vi "Acquire_Prototype.vi"() -> ()   [LabVIEW 2013, in "MagSpec_Bella.lvclass"]
uses:
  MagSpec_Bella.lvclass
  Controls/CamAndObj_TypDEf_Bella.ctl
  Controls/ScreenCam2_TypDEf_Bella.ctl
  MagSpec_Bella.lvclass/MagSpec_Bella.ctl
  <vilib>/vision/NI_Vision_Development_Module.lvlib
panel:
  out "get Images":u32
  out "Array 3":i32[][](array[numeric])
  out "Array 2":i32[][](array[numeric])
  out "time":u32[](array[numeric])
  out "total time":u32
  out "B":dbl
  in  "Sim Image Index 2":i32=3
  in  "B [T] in":dbl=0.63
  out "Numeric 3":i32
  in  "stop":bool
  out "Image Out":T1(plugin-control)
  out "Empty Image":bool[](array[boolean])
  out "error out":errorcluster
  out "Sum Y":cluster{"Momentum [MeV/C]":dbl[], dbl[]}[](graph)
  in  "MagSpec_Bella.lvclass":refnum<class "MagSpec_Bella.lvclass">
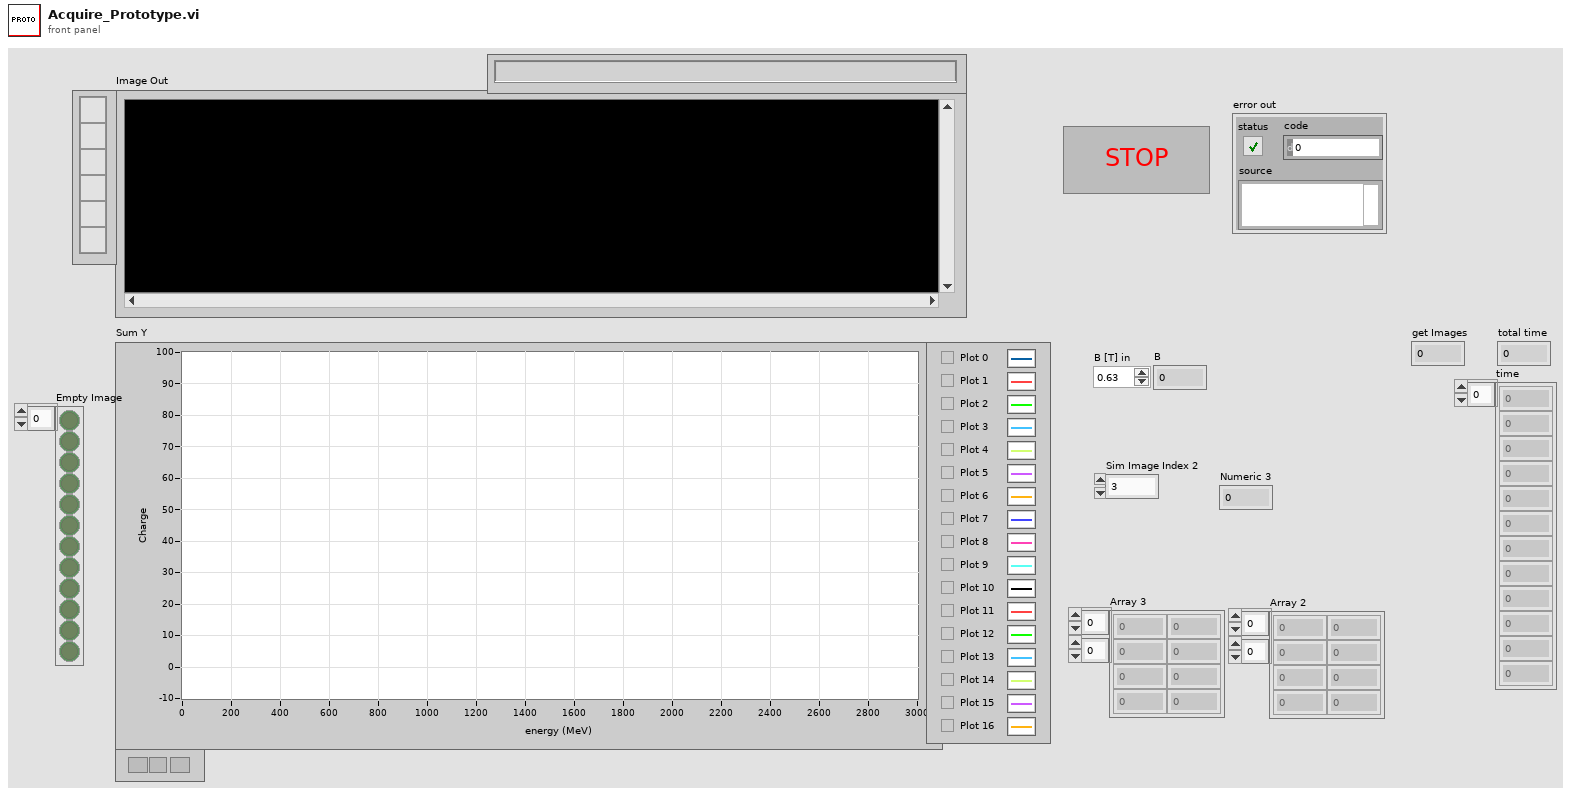
[diagram p1: front panel]
types:
  T1 = typedef "IMAQ Image.ctl" = refnum<image>
  T2 = typedef "Image Type" = u32
  T3 = typedef "CameraSettings_File.ctl" = cluster{"FOV [mm]":dbl, "Left edge [mm]":dbl, "ROI Y offset":dbl, "ROI height":dbl, "ROI X offset":dbl, "ROI width":dbl, "Y center pixel":dbl, "Y Start":dbl, "Y End":dbl, "X Start":dbl, "X End":dbl, "rot [deg]":dbl}
  T4 = typedef "ScreenCam2_TypDEf_Bella.ctl" = cluster{"Screen Orientation":string, "Screen angle":string, "Lens":T5, "Calibration (mm/pix)":dbl}
  T5 = typedef "CamAndObj_TypDEf_Bella.ctl" = enum16{"FL1-f8x08", "FL1-f8x06", "FL1-f8", "ch300-f50", "FL2G-f8", "FL3M14-f8", "FL3M14-f8x08", "FL3M14-f8x08(2x2)"}
  T6 = cluster{"npix-X":i32, "npix-Y":i32, "Left [pix]":dbl, "Top [pix]":dbl}
  T7 = typedef "OneTimeCalculation.ctl" = cluster{"first Pixel pos [m]":dbl, "Pixel Size [mm]":dbl, "forward":T8}
  T8 = typedef "OnOffTypeDef.ctl" = enum16{"off", "on"}
  T9 = typedef "2D.ctl" = cluster{"dp":dbl[][], "chargeCompensation":dbl[][], "angle":dbl[][], "Momentum":dbl[][]}
  T10 = typedef "finalCalib--Cluster.ctl" = cluster{"X":dbl[][], "xi":dbl[][], "delta momentum":dbl, "Y":dbl[][], "yi":dbl[][], "angle (Y)":dbl[], "delta angle":dbl, "scale delta angle":dbl, "intraX":dbl, "intraY":dbl, "mask":dbl[][]}
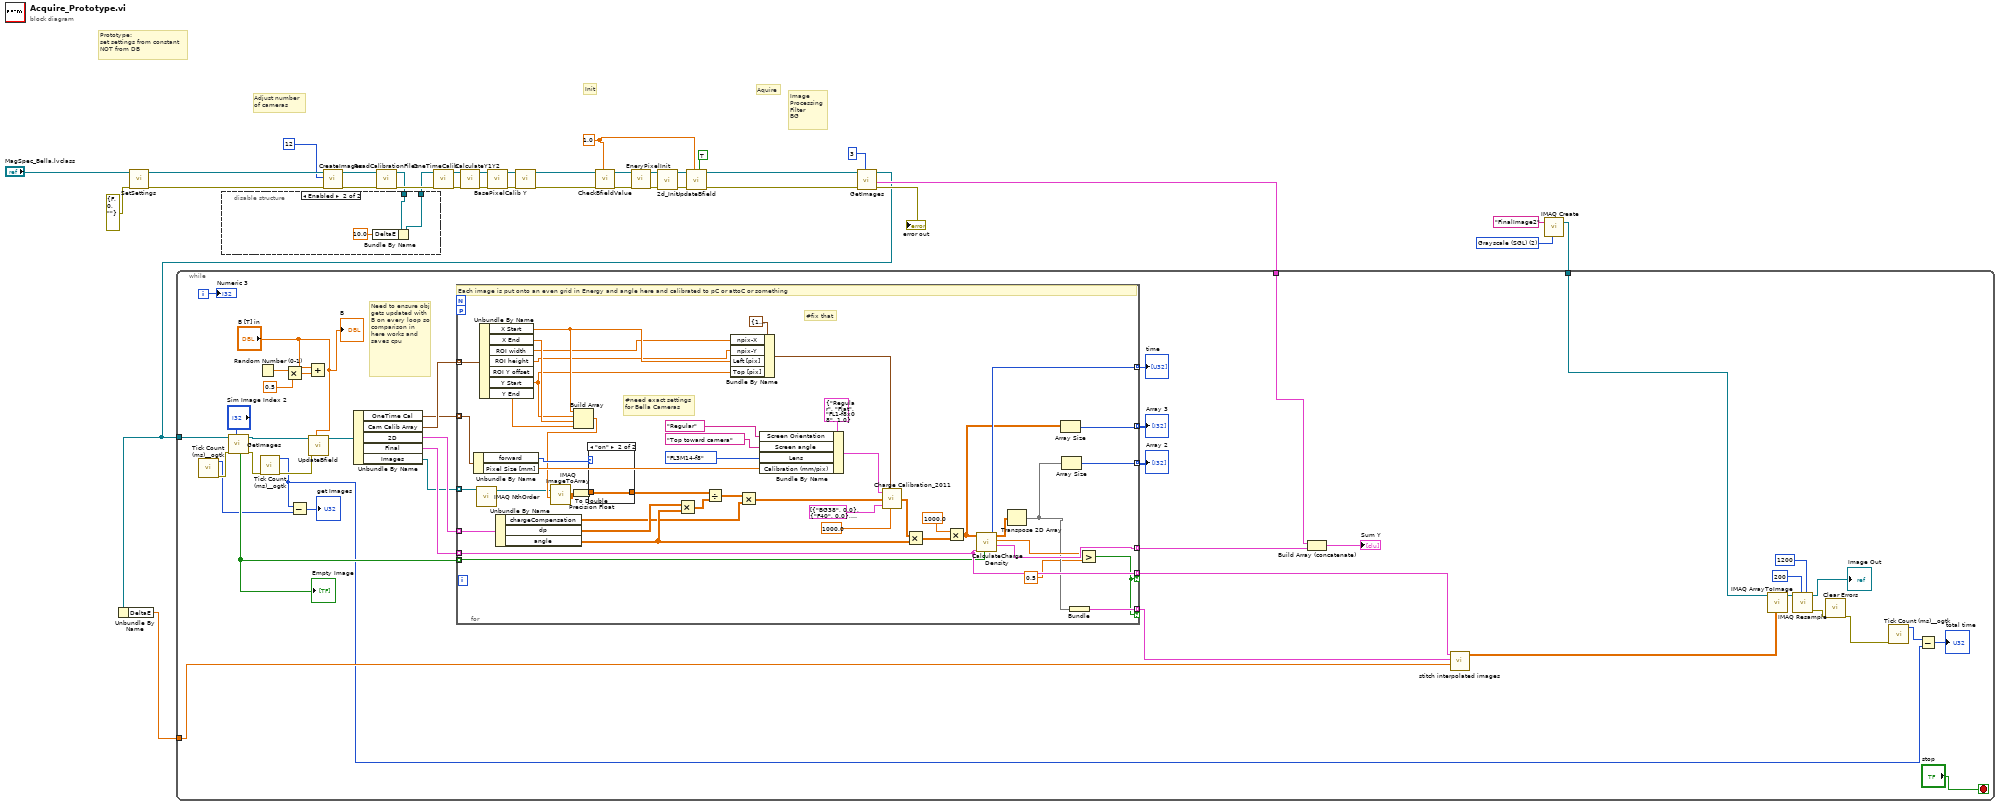
[diagram p0: block diagram]
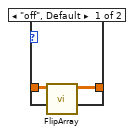
[diagram p2: hidden frame]
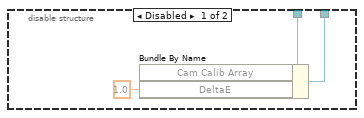
[diagram p3: hidden frame]
diagram:
  w3 = 1.0 ("B [T] in")
  w7 = T2 2 items=["Grayscale (U8)", "Grayscale (I16)", "Grayscale (SGL)", "Complex (CSG)", "RGB (U32)", "HSL (U32)", "RGB (U64)", "Grayscale (U16)"] ("Image Type")
  # "Image\nProcessing\nFilter\nBG"
  # "Adjust number\nof cameras"
  # "Aquire"
  # "Init"
  # "Prototype:\nset settings from constant\nNOT from DB"
  n1 = call "SetSettings.vi"("error in (no error)"=errorcluster {"status"=FALSE, "code"=0, "source"=""} ("error out"), "MagSpec_Bella in"="MagSpec_Bella.lvclass") -> ("error out"=w31:errorcluster, "MagSpec_Bella out"=w33:refnum<class "MagSpec_Bella.lvclass">)  [unwired: 8 in]
  n2 = call "CreateImages.vi"("error in (no error)"=w31, "Numeric"=12, "MagSpec_Bella in"=w33) -> ("error out"=w30:errorcluster, "MagSpec_Bella out"=w15:refnum<class "MagSpec_Bella.lvclass">)  [unwired: 7 in]
  n3 = call "ReadCalibrationFiles.vi"("error in (no error)"=w30, "MagSpec_Bella in"=w15) -> ("error out"=w29:errorcluster, "MagSpec_Bella out"=w14:refnum<class "MagSpec_Bella.lvclass">)  [unwired: 8 in]
  n4 = disable-structure shown="Enabled" {
    disable-tunnel: w14 -> [w38 w42]
    disable-tunnel: [w37 w41] -> w13
    frame Disabled {
      n5 = Bundle By Name(cluster=w38, "DeltaE"=1.0) -> (w37:refnum<class "MagSpec_Bella.lvclass">, "Cam Calib Array"=w39:T3[])
    }
    frame Enabled {
      n6 = Bundle By Name(cluster=w42, "DeltaE"=10.0) -> (w41:refnum<class "MagSpec_Bella.lvclass">)
    }
  }
  n7 = call "OneTimeCalib.vi"("error in"=w29, "MagSpec_Bella in"=w13) -> ("error out"=w24:errorcluster, "MagSpec_Bella out"=w25:refnum<class "MagSpec_Bella.lvclass">)  [unwired: 8 in]
  n8 = call "CalculateY1Y2.vi"("error in"=w24, "MagSpec_Bella in"=w25) -> ("error out"=w22:errorcluster, "MagSpec_Bella out"=w23:refnum<class "MagSpec_Bella.lvclass">)  [unwired: 8 in]
  n9 = call "BasePixelCalib.vi"("error in (no error)"=w22, "MagSpec_Bella in"=w23) -> ("error out"=w19:errorcluster, "MagSpec_Bella out"=w21:refnum<class "MagSpec_Bella.lvclass">)  [unwired: 8 in]
  n10 = call "Y.vi"("error in (no error)"=w19, "MagSpec_Bella in"=w21) -> ("error out"=w18:errorcluster, "MagSpec_Bella out"=w20:refnum<class "MagSpec_Bella.lvclass">)  [unwired: 8 in]
  n11 = call "CheckBfieldValue .vi"("B [T] new"=w3, "MagSpec_Bella in"=w20) -> ("MagSpec_Bella out"=w8:refnum<class "MagSpec_Bella.lvclass">)  [unwired: 8 in, 1 out]
  n12 = call "EneryPixelInit.vi"("error in (no error)"=w18, "MagSpec_Bella in"=w8) -> ("error out"=w9:errorcluster, "MagSpec_Bella out"=w10:refnum<class "MagSpec_Bella.lvclass">)  [unwired: 8 in]
  n13 = call "2d_Init.vi"("error in (no error)"=w9, "MagSpec_Bella in"=w10) -> ("error out"=w26:errorcluster, "MagSpec_Bella out"=w27:refnum<class "MagSpec_Bella.lvclass">)  [unwired: 8 in]
  n14 = call "UpdateBfield.vi"("Force upodate (F)"=TRUE ("Force upodate"), "B [T] in"=w3, "error in (no error)"=w26, "MagSpec_Bella in"=w27) -> ("error out"=w28:errorcluster, "MagSpec_Bella out"=w35:refnum<class "MagSpec_Bella.lvclass">)  [unwired: 6 in]
  n15 = call "GetImages.vi"("Sim Image Index"=3, "error in (no error)"=w28, "MagSpec_Bella in"=w35) -> ("error out"=→"error out":errorcluster, "output cluster"=w12:cluster{dbl[], dbl[]}[], "MagSpec_Bella out"=w2:refnum<class "MagSpec_Bella.lvclass">)  [unwired: 5 in, 1 out]
  n16 = Unbundle By Name(w2) -> ("DeltaE"=w1:dbl)
  n17 = call "IMAQ Create"("Image Name"="FinalImage2", "Image Type"=w7) -> ("New Image"=w5:T1)  [unwired: 3 in, 1 out]
  n18 = while {
    tunnel: w12 -> [w78]
    tunnel: w5 -> [w77]
    tunnel: w2 -> [w66]
    tunnel: w1 -> [w60]
    i -> [w71]
    stop <- "stop" stop-if-true
    # "Need to ensure obj gets updated with B on every loop so comparison in here works and saves cpu"
    n19 = call <userlib>:"Tick Count (ms)__ogtk.vi"() -> ("error out"=w46:errorcluster, "millisecond timer value"=w44:u32)  [unwired: 10 in]
    n20 = call "GetImages.vi"("Sim Image Index"="Sim Image Index 2", "error in (no error)"=w46, "MagSpec_Bella in"=w66) -> ("error out"=w48:errorcluster, "MagSpec_Bella out"=w65:refnum<class "MagSpec_Bella.lvclass">, "Empty Image"=w58:bool[])  [unwired: 5 in, 1 out]
    "Empty Image" <- w58
    n21 = Random Number (0-1)() -> (number: 0 to 1=w70:dbl)
    n22 = call <userlib>:"Tick Count (ms)__ogtk.vi"("error in (no error)"=w48) -> ("error out"=w47:errorcluster, "millisecond timer value"=w45:u32)  [unwired: 9 in]
    n23 = Multiply(x=w70, y=0.5) -> (x*y=w68:dbl)
    n24 = Subtract(x=w45, y=w44) -> (x-y=→"get Images":u32)
    n25 = Add(x="B [T] in", y=w68) -> ()  [unwired: 1 out]
    n26 = call "UpdateBfield.vi"("B [T] in"="B [T] in", "error in (no error)"=w47, "MagSpec_Bella in"=w65) -> ("MagSpec_Bella out"=w73:refnum<class "MagSpec_Bella.lvclass">)  [unwired: 7 in, 1 out]
    n27 = Unbundle By Name(w73) -> ("OneTime Cal"=w79:T7[], "Cam Calib Array"=w80:T3[], "2D"=w83:T9[], "Final"=w82:T10[], "Images"=w81:T1[])
    n28 = for {
      tunnel: w83 -> [w131] mode=indexing
      tunnel: w82 -> [w96] mode=indexing
      tunnel: w81 -> [w116] mode=indexing
      tunnel: w80 -> [w129] mode=indexing
      tunnel: w79 -> [w128] mode=indexing
      tunnel: [w117] -> w76 mode=indexing
      tunnel: [w96] -> w75 mode=indexing if=w93
      tunnel: [w95] -> w74 mode=indexing if=w93
      workers-P: _ -> [_]
      tunnel: w58 -> [w90] mode=indexing
      tunnel: [w89] -> w49 mode=indexing
      tunnel: [w87] -> w62 mode=indexing
      tunnel: [w85] -> w61 mode=indexing
      # "#fix that"
      # "#need exact settings\nfor Bella Cameras"
      # "Each image is put onto an even grid in Energy and angle here and calibrated to pC or attoC or something"
      n29 = Unbundle By Name(w128) -> ("forward"=w103:T8, "Pixel Size [mm]"=w127:dbl)
      n30 = call "IMAQ NthOrder"("Image Src"=w116) -> ("Image Dst Out"=w101:T1)  [unwired: 6 in, 1 out]
      n31 = Unbundle By Name(w129) -> ("X Start"=w107:dbl, "X End"=w112:dbl, "ROI width"=w105:dbl, "ROI height"=w104:dbl, "Y Start"=w106:dbl, "Y End"=w111:dbl)  [unwired: 1 out]
      n32 = Unbundle By Name(w131) -> ("chargeCompensation"=w114:dbl[][], "dp"=w115:dbl[][], "angle"=w130:dbl[][])
      n33 = Build Array(w107, w106, w112, w111) -> (w102:dbl[])
      n34 = call "IMAQ ImageToArray"("Optional Rectangle"=w102, "Image"=w101) -> ("Image Pixels (Float)"=w97:sgl[][])  [unwired: 2 in, 4 out]
      n35 = To Double Precision Float(number=w97) -> (double precision float=w109:dbl[][])
      n36 = case shown="\"on\"" w103 {
        tunnel: w109 -> [w133 w134]
        tunnel: [w132 w134] -> w108
        frame "off", Default {
          n37 = call "FlipArray.vi"("In"=w133) -> ("Out"=w132:dbl[][])  [unwired: 10 in]
        }
        frame "on" {
        }
      }
      n38 = Multiply(x=w115, y=w130) -> (x*y=w92:dbl[][])
      n39 = Divide(x=w108, y=w92) -> (x/y=w91:dbl[][])
      n40 = Bundle By Name(cluster=T6 {"npix-X"=1384, "npix-Y"=300, "Left [pix]"=0.0, "Top [pix]"=0.0} ("ROI infos"), "npix-X"=w105, "npix-Y"=w104, "Left [pix]"=w107, "Top [pix]"=w106) -> (w98:T6)
      n41 = Multiply(x=w91, y=w114) -> (x*y=w113:dbl[][])
      n42 = Bundle By Name(cluster=T4 {"Screen Orientation"="Regular", "Screen angle"="Flat", "Lens"=enum."FL1-f8x08", "Calibration (mm/pix)"=1.0} ("Screen&Camera 2"), "Screen Orientation"="Regular", "Screen angle"="Top toward camera", "Lens"=CamAndObj_TypDEf_Bella."FL3M14-f8", "Calibration (mm/pix)"=w127) -> (w122:T4)
      n43 = call "Charge Calibration_2011.vi"("Screen&Camera 2"=w122, "ROI infos"=w98, "Image (Counts)"=w113, "Filters"=cluster{"Name":string, "#Filters":dbl}[] [{"Name"="BG38", "#Filters"=0.0}, {"Name"="F40", "#Filters"=0.0}, {"Name"="F70", "#Filters"=1.0}, {"Name"="oldBP", "#Filters"=0.0}], "Electron energy (MeV)"=1000.0) -> ("Image (pC)"=w120:dbl[][])  [unwired: 4 in]
      n44 = Multiply(x=w120, y=w130) -> (x*y=w100:dbl[][])
      n45 = Multiply(x=1000.0, y=w100) -> (x*y=w86:dbl[][])
      n46 = call "CalculateChargeDensity.vi"("empty image"=w90, "Final"=w96, "Z"=w86) -> ("spec cluster 2"=w117:cluster{"Momentum [MeV/C]":dbl[], dbl[]}, "charge (sum)"=w94:dbl, "charge density"=w118:dbl[][], "time: 2Dinter"=w89:u32)  [unwired: 4 in, 1 out]
      n47 = Transpose 2D Array(2D array=w118) -> (transposed array=w88:dbl[][])
      n48 = Array Size(array=w86) -> (size(s)=w85:i32[])
      n49 = Array Size(array=w88) -> (size(s)=w87:i32[])
      n50 = Bundle(w88) -> (w95:cluster{dbl[][]})  [unwired: 1 in]
      n51 = Greater?(x=w94, y=0.5 ("change threshold")) -> (0:w93:bool)
    }
    "time" <- w49
    "Array 2" <- w62
    "Array 3" <- w61
    n52 = Build Array (concatenate)(w78, w76) -> (→"Sum Y":cluster{"Momentum [MeV/C]":dbl[], dbl[]}[])
    n53 = call "stitch interpolated images.vi"("DeltaE"=w60, "Array of images to stitch"=w74, "calib \"final\""=w75) -> ("stitched array image"=w55:sgl[][])  [unwired: 8 in]
    n54 = call "IMAQ ArrayToImage"("Image Pixels (Float)"=w55, "Image"=w77) -> ("Image Out"=w54:T1)  [unwired: 8 in, 1 out]
    n55 = call "IMAQ Resample"("X Resolution"=1200, "Y Resolution"=200, "Image Src"=w54) -> ("error out"=w51:errorcluster, "Image Dst Out"=→"Image Out":T1)  [unwired: 7 in]
    n56 = call <vilib>:"Clear Errors.vi"("error in (no error)"=w51) -> ("error out"=w63:errorcluster)  [unwired: 6 in]
    n57 = call <userlib>:"Tick Count (ms)__ogtk.vi"("error in (no error)"=w63) -> ("millisecond timer value"=w57:u32)  [unwired: 9 in, 1 out]
    n58 = Subtract(x=w57, y=w45) -> (x-y=→"total time":u32)
    "Numeric 3" <- w71
    "B" <- "B [T] in"
  }
